vi "String - Value Change.vi"(8 "error in (no error)":errorcluster, 11 "Loop data in":T1={"Config"={"List"=[], "max rows"=8, "Listbox placement"=enum."None", "String Color Options"={"Use? (F)"=FALSE, "Color - Valid"=0, "Color - Invalid"=0, "Allow blank?"=FALSE}}, "Refs"={"String"=refnum, "Listbox"=refnum}, "State"={"LB active?"=FALSE}}) -> (0 "error out":errorcluster, 3 "Loop data out":T1={"Config"={"List"=[], "max rows"=8, "Listbox placement"=enum."None", "String Color Options"={"Use? (F)"=FALSE, "Color - Valid"=0, "Color - Invalid"=0, "Allow blank?"=FALSE}}, "Refs"={"String"=refnum, "Listbox"=refnum}, "State"={"LB active?"=FALSE}})   [LabVIEW 2021, in "Autocomplete Textbox.lvlib"]
uses:
  Autocomplete Textbox.lvlib
  Loop Data.ctl
  Inputs.ctl
  Classes/Handle/Listbox placement.ctl
  Color String Options.ctl
  Refs.ctl
  State data.ctl
  Classes/Handle/Handle.lvclass
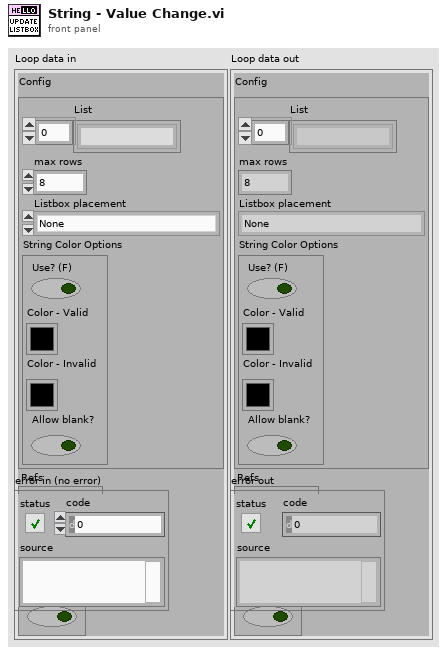
[diagram p1: front panel]
types:
  T1 = typedef "Autocomplete Textbox.lvlib/Loop Data.ctl" = cluster{"Config":T2, "Refs":T5, "State":T6}
  T2 = typedef "Autocomplete Textbox.lvlib/Inputs.ctl" = cluster{"List":string[], "max rows":i32, "Listbox placement":T3, "String Color Options":T4}
  T3 = typedef "Autocomplete Textbox.lvlib/Handle.lvclass/Listbox placement.ctl" = enum16{"None", "Under String", "Fit to Pane"}
  T4 = typedef "Autocomplete Textbox.lvlib/Color String Options.ctl" = cluster{"Use? (F)":bool, "Color - Valid":u32, "Color - Invalid":u32, "Allow blank?":bool}
  T5 = typedef "Autocomplete Textbox.lvlib/Refs.ctl" = cluster{"String":refnum<vi>, "Listbox":refnum<vi>}
  T6 = typedef "Autocomplete Textbox.lvlib/State data.ctl" = cluster{"LB active?":bool}
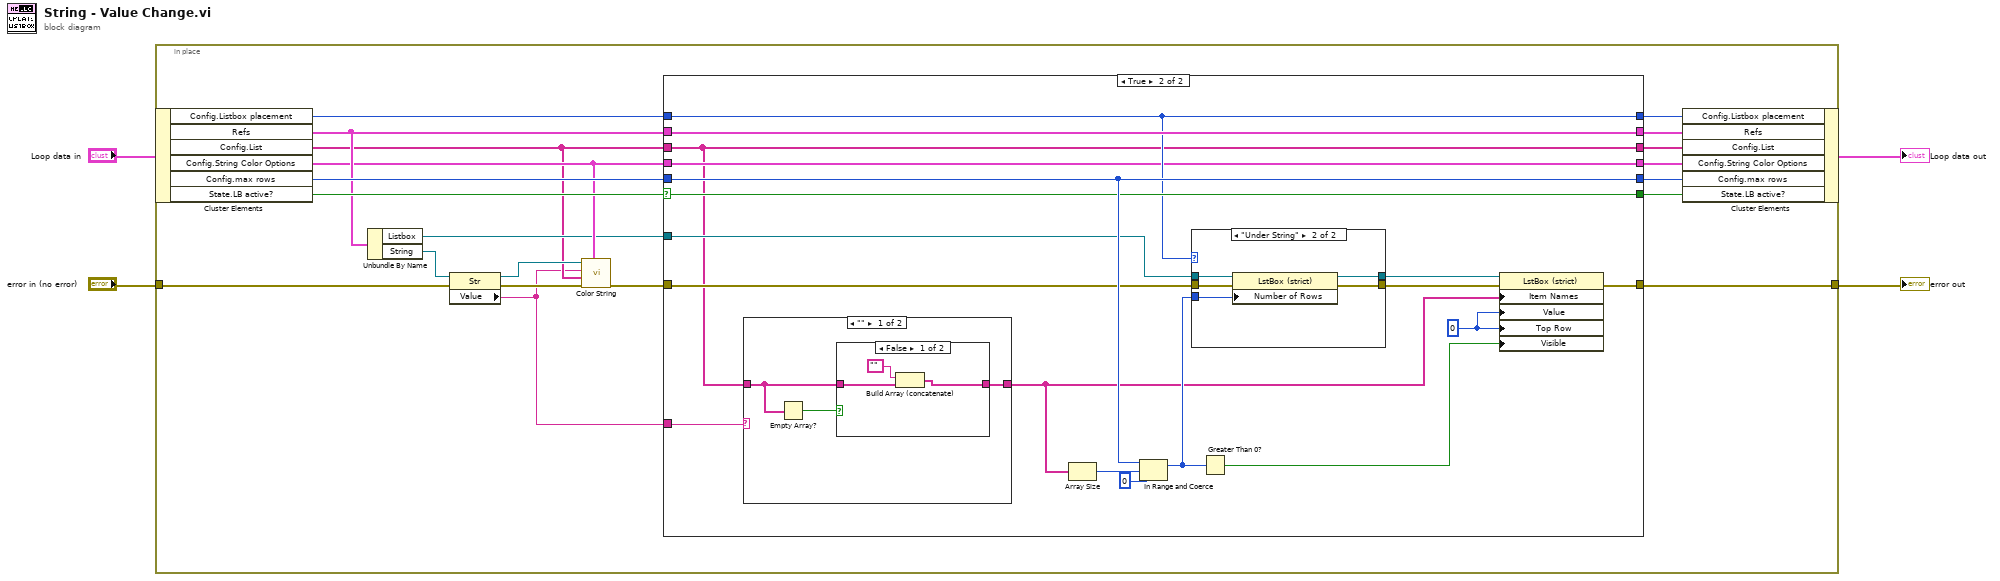
[diagram p0: block diagram]
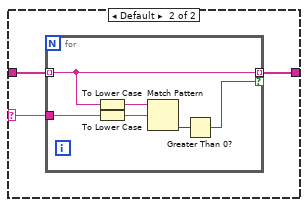
[diagram p4: hidden frame]
diagram:
  n1 = in-place {
    in-place-border: "error in (no error)" -> [w13]
    in-place-border: [w23] -> w1
    n2 = in-place-cluster #1("Loop data in") -> ("Config.Listbox placement"=w17:T3, "Refs"=w14:T5, "Config.List"=w6:string[], "Config.String Color Options"=w10:T4, "Config.max rows"=w24:i32, "State.LB active?"=w22:bool)
    n3 = Unbundle By Name(w14) -> ("Listbox"=w7:refnum<vi>, "String"=w15:refnum<vi>)
    n4 = property class="Str"(reference=w15, error in=w13) -> (reference out=w11:refnum<vi>, error out=w12:errorcluster, "Value"=w5:string)
    n5 = call "Color String.vi"("Options"=w10, "error in (no error)"=w12, "Config.List"=w6, "String.Value"=w5, "String"=w11) -> ("error out"=w8:errorcluster)  [unwired: 6 in]
    n6 = case shown="True" w22 {
      selector: w22 -> [w28 w43]
      tunnel: w6 -> [w30 w34]
      tunnel: w24 -> [w29 w44]
      tunnel: [w27 w46] -> w23
      tunnel: w14 -> [w31 w45]
      tunnel: w8 -> [w27 w36]
      tunnel: [w31 w45] -> w21
      tunnel: [w30 w34] -> w20
      tunnel: [w29 w44] -> w19
      tunnel: [w28 w43] -> w18
      tunnel: w17 -> [w26 w40]
      tunnel: [w26 w40] -> w16
      tunnel: w10 -> [w25 w38]
      tunnel: [w25 w38] -> w9
      tunnel: w7 -> [_ w37]
      tunnel: w5 -> [_ w33]
      frame False {
      }
      frame True {
        w47 = 0 ("Value")
        n7 = case shown="\"\"" w33 {
          selector: w33 -> [_ w58]
          tunnel: w34 -> [w51 w59]
          tunnel: [w52 w57] -> w35
          frame "" {
            n8 = Empty Array?(array=w51) -> (empty?=w50:bool)
            n9 = case shown="False" w50 {
              tunnel: [w54 w56] -> w52
              tunnel: w51 -> [w53 w56]
              frame False {
                n10 = Build Array (concatenate)("", w53) -> (w54:string[])
              }
              frame True {
              }
            }
          }
          frame Default {
            n11 = for {
              tunnel: w59 -> [w63] mode=indexing
              tunnel: w58 -> [w61]
              tunnel: [w63] -> w57 mode=indexing if=w64
              n12 = To Lower Case(string=w63) -> (all lower case string=w62:string)
              n13 = To Lower Case(string=w61) -> (all lower case string=w60:string)
              n14 = Match Pattern(string=w62, regular expression=w60) -> (offset past match=w65:i32)  [unwired: 1 in, 3 out]
              n15 = Greater Than 0?(x=w65) -> (x > 0?=w64:bool)
            }
          }
        }
        n16 = Array Size(array=w35) -> (size(s)=w49:i32)
        n17 = In Range and Coerce(upper limit=w44, x=w49, lower limit=0) -> (coerced(x)=w39:i32)  [unwired: 1 out]
        n18 = case shown="\"Under String\"" w40 {
          tunnel: w37 -> [w67 w72]
          tunnel: [w67 w71] -> w42
          tunnel: [w66 w70] -> w41
          tunnel: w39 -> [_ w69]
          tunnel: w36 -> [w66 w68]
          frame "None", "Fit to Pane" {
          }
          frame "Under String" {
            n19 = property on="Property Node" class="LstBox (strict)"(reference=w72, error in=w68, "Number of Rows"=w69) -> (reference out=w71:refnum<vi>, error out=w70:errorcluster)
          }
        }
        n20 = Greater Than 0?(x=w39) -> (x > 0?=w32:bool)
        n21 = property on="Property Node" class="LstBox (strict)"(reference=w42, error in=w41, "Item Names"=w35, "Value"=w47, "Top Row"=w47, "Visible"=w32) -> (error out=w46:errorcluster)  [unwired: 1 out]
      }
    }
    n22 = in-place-cluster #1("Config.Listbox placement"=w16, "Refs"=w21, "Config.List"=w20, "Config.String Color Options"=w9, "Config.max rows"=w19, "State.LB active?"=w18) -> (→"Loop data out":T1)
  }
  "error out" <- w1
